vi "pass_pipe.vi"(7 "bird":sgl, 8 "error in (no error)":errorcluster, 9 "y lower":sgl, 10 "y upper":sgl) -> (0 "error out":errorcluster, 2 "pass":bool)   [LabVIEW 2017]
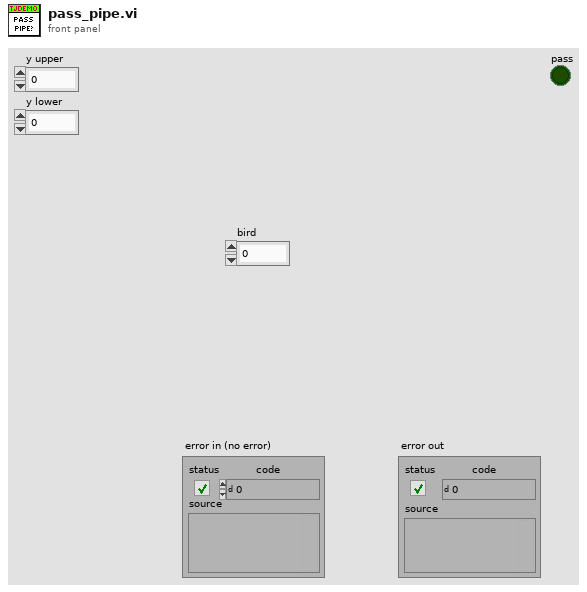
[diagram p1: front panel]
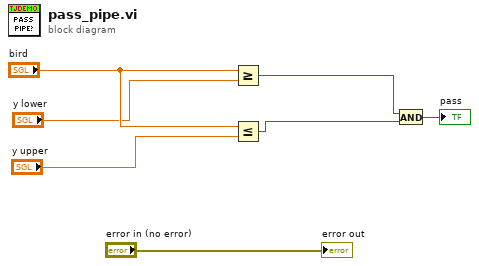
[diagram p0: block diagram]
diagram:
  n1 = Greater Or Equal?(x="bird", y="y lower") -> (x >= y?=w4:bool)
  n2 = Less Or Equal?(x="bird", y="y upper") -> (x <= y?=w3:bool)
  n3 = And(x=w4, y=w3) -> (x .and. y?=→"pass":bool)
  "error out" <- "error in (no error)"
